vi "Convert RAWDATA_Denis.vi"(0 "Detector in":refnum<class "Detector.lvclass">, 1 "I channel":sgl[][](array[numeric]), 3 "WCM_values IN":sgl[](array[numeric]), 4 "II channel":sgl[][](array[numeric]), 5 "error in (no error)":errorcluster, 6 "# of scan":i32, 7 "All?":bool=TRUE, 10 "repump_limits":T1, 11 "repump_correction":bool, 12 "I channel seq IN":cluster{"BG":sgl[], "Ie":sgl[], "I0":sgl[]}[](array[cluster]), 13 "II channel seq IN":cluster{"BG":sgl[], "Ie":sgl[], "I0":sgl[]}[](array[cluster])) -> (14 "Detector out":refnum<class "Detector.lvclass">, 15 "I channel seq":cluster{"BG":sgl[], "Ie":sgl[], "I0":sgl[]}[](array[cluster]), 17 "WCM_correction_coff":sgl[](array[numeric]), 18 "II channel seq":cluster{"BG":sgl[], "Ie":sgl[], "I0":sgl[]}[](array[cluster]), 19 "error out":errorcluster)   [LabVIEW 2020, in "Detector.lvclass"]
uses:
  Detector.lvclass
  <userlib>/_OpenG.lib/array/array.llb/Search 1D Array (SGL)__ogtk.vi
  dependecies/globalVarII.vi
  dependecies/ControlsVIs/Clusters-def/Def_repump_limits.ctl
  Oscilloscope/Oscilloscope.lvclass
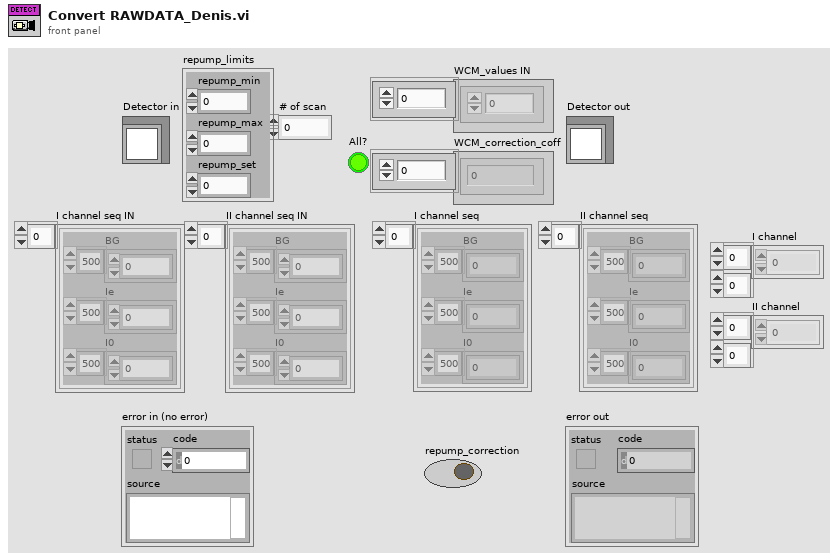
[diagram p1: front panel]
types:
  T1 = typedef "Oscilloscope.lvclass/Def_repump_limits.ctl" = cluster{"repump_min":dbl, "repump_max":dbl, "repump_set":dbl}
  T2 = typedef "Control-Client.lvclass/Controls-refs_CLIENT.ctl" = cluster{"ON/OFF Cool":refnum<vi>, "Save spectra":refnum<vi>, "Read detector":refnum<vi>, "# scans":refnum<vi>, "BG-level":refnum<vi>, "Set T":refnum<vi>, "Termometer":refnum<vi>, "Spectra":refnum<vi>, "Error Meter_ref":refnum<vi>, "OD graph":refnum<vi>, "from_pixel":refnum<vi>, "to_pixel":refnum<vi>, "threshold_ref_channel":refnum<vi>, "value":refnum<vi>, "python session":refnum<vi>, "ref h5_file":T3, "distance":refnum<vi>}
  T3 = typedef "hid_t.ctl" = i64
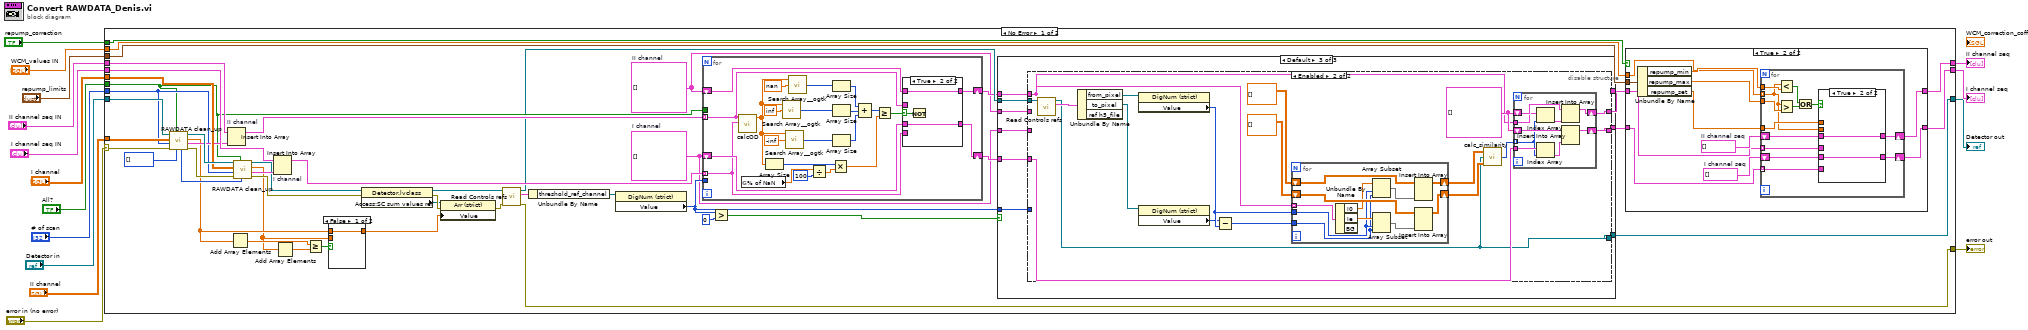
[diagram p0: block diagram]
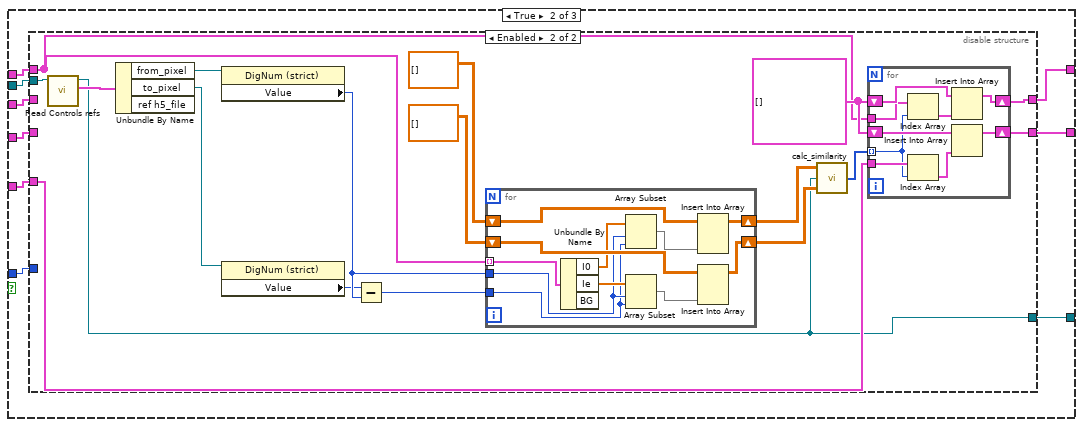
[diagram p3: hidden frame]
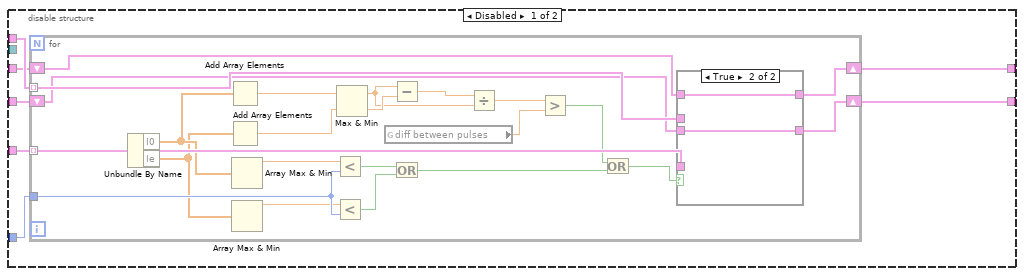
[diagram p4: hidden frame]
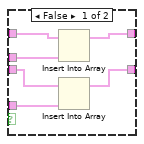
[diagram p5: hidden frame]
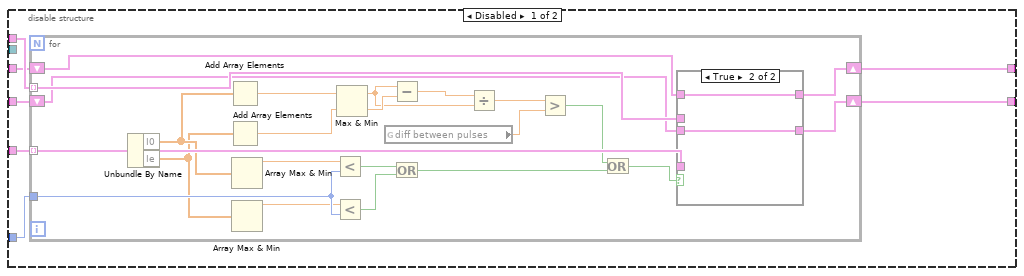
[diagram p6: hidden frame]
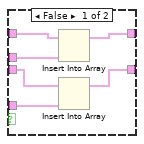
[diagram p7: hidden frame]
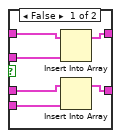
[diagram p8: hidden frame]
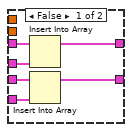
[diagram p11: hidden frame]
diagram:
  n1 = case shown="No Error" "error in (no error)" {
    selector: "error in (no error)" -> [w55 w306]
    tunnel: [w16 w307] -> w12
    tunnel: "Detector in" -> [w54 w307]
    tunnel: [w17 w306] -> w11
    tunnel: [w62 w305] -> w15
    tunnel: [w61 w304] -> w14
    tunnel: "II channel seq IN" -> [w60 w305]
    tunnel: "I channel seq IN" -> [w59 w304]
    tunnel: "WCM_values IN" -> [w58 _]
    tunnel: "I channel" -> [w44 _]
    tunnel: "II channel" -> [w46 _]
    tunnel: "repump_correction" -> [w57 _]
    tunnel: "repump_limits" -> [w56 _]
    tunnel: "All?" -> [w30 _]
    tunnel: "# of scan" -> [w37 _]
    frame No Error {
      w20 = cluster{"BG":sgl[], "Ie":sgl[], "I0":sgl[]}[] []  # II channel
      w21 = cluster{"BG":sgl[], "Ie":sgl[], "I0":sgl[]}[] []  # I channel
      n2 = call "RAWDATA clean_up.vi"("BG index IN"=i32[] [], "All?"=w30, "error in (no error)"=w55, "# of scan"=w37, "channel"=w46, "Detector in"=w54) -> ("error out"=w48:errorcluster, "channel seq"=w42:cluster{"BG":i32[], "Ie":i32[], "I0":i32[]}[], "SC values"=w38:sgl[], "Detector out"=w47:refnum<class "Detector.lvclass">, "BG indexes"=w45:i32[])  [unwired: 1 in]
      n3 = Insert Into Array "II channel"(array=w60, new element=w42) -> (w34:cluster{"BG":sgl[], "Ie":sgl[], "I0":sgl[]}[])  [unwired: 1 in]
      n4 = Add Array Elements(numeric array=w38) -> (sum=w51:sgl)
      n5 = call "RAWDATA clean_up.vi"("BG index IN"=w45, "All?"=w30, "error in (no error)"=w48, "# of scan"=w37, "channel"=w44, "Detector in"=w47) -> ("error out"=w40:errorcluster, "channel seq"=w43:cluster{"BG":i32[], "Ie":i32[], "I0":i32[]}[], "SC values"=w31:sgl[], "Detector out"=w41:refnum<class "Detector.lvclass">)  [unwired: 1 in, 1 out]
      n6 = Insert Into Array "I channel"(array=w59, new element=w43) -> (w35:cluster{"BG":sgl[], "Ie":sgl[], "I0":sgl[]}[])  [unwired: 1 in]
      n7 = Add Array Elements(numeric array=w31) -> (sum=w50:sgl)
      n8 = Greater Or Equal?(x=w51, y=w50) -> (x >= y?=w49:bool)
      n9 = case shown="False" w49 {
        tunnel: w38 -> [w268 _]
        tunnel: [w268 w269] -> w39
        tunnel: w31 -> [_ w269]
        frame False {
        }
        frame True {
        }
      }
      n10 = property class="Detector.lvclass"(reference=w41, error in=w40) -> (reference out=w28:refnum<class "Detector.lvclass">, error out=w53:errorcluster, "Access:SC sum values ref"=w52:refnum<vi>)
      n11 = property class="Arr (strict)"(reference=w52, error in=w53, "Value"=w39) -> (error out=w29:errorcluster)  [unwired: 1 out]
      n12 = call "Read Controls refs.vi"("error in (no error)"=w29, "Detector in"=w28) -> ("error out"=w17:errorcluster, "Controls refs"=w27:T2, "Detector out"=w24:refnum<class "Detector.lvclass">)  [unwired: 7 in]
      n13 = Unbundle By Name(w27) -> ("threshold_ref_channel"=w26:refnum<vi>)
      n14 = property class="DigNum (strict)"(reference=w26) -> ("Value"=w25:i32)  [unwired: 1 in, 2 out]
      n15 = for {
        tunnel: w35 -> [w238] mode=indexing
        tunnel: w34 -> [w248] mode=indexing
        shift-right: [w236] -> w22
        shift-left: w21 -> [w250]
        shift-right: [w237] -> w23
        shift-left: w20 -> [w249]
        tunnel: w30 -> [_]
        tunnel: w25 -> [_]
        n16 = call "calcOD.vi"("channel I"=w238, "channel 2"=w248) -> ("OD"=w256:sgl[])  [unwired: 3 in, 6 out]
        n17 = global read "globalVarII.vi" "% of NaN"() -> (w246:sgl)
        n18 = Array Size(array=w256) -> (size(s)=w255:i32)
        n19 = call-poly <userlib>:"Search Array__ogtk.vi"("Array"=w256, "Element Data"=sgl inf) -> ("Indices of Elements"=w254:i32[])  [unwired: 7 in]
        n20 = call-poly <userlib>:"Search Array__ogtk.vi"("Array"=w256, "Element Data"=sgl -inf) -> ("Indices of Elements"=w253:i32[])  [unwired: 7 in]
        n21 = call-poly <userlib>:"Search Array__ogtk.vi"("Array"=w256, "Element Data"=sgl nan) -> ("Indices of Elements"=w257:i32[])  [unwired: 7 in]
        n22 = Divide(x=w246, y=100) -> (x/y=w247:sgl)
        n23 = Multiply(x=w255, y=w247) -> (x*y=w240:sgl)
        n24 = Array Size(array=w257) -> (size(s)=w244:i32)
        n25 = Array Size(array=w254) -> (size(s)=w243:i32)
        n26 = Array Size(array=w253) -> (size(s)=w242:i32)
        n27 = Compound Arithmetic op=ADD(w244, w243, w242) -> (w241:i32)
        n28 = Greater Or Equal?(x=w241, y=w240) -> (x >= y?=w239:bool)
        n29 = case shown="True" w239 {
          selector: w239 -> [_ w265]
          tunnel: w250 -> [w264 w266]
          tunnel: w238 -> [w263 _]
          tunnel: [w262 w266] -> w236
          tunnel: [w261 w267] -> w237
          tunnel: w249 -> [w260 w267]
          tunnel: w248 -> [w259 _]
          frame False {
            n30 = Insert Into Array(array=w260, new element=w259) -> (w261:cluster{"BG":sgl[], "Ie":sgl[], "I0":sgl[]}[])  [unwired: 1 in]
            n31 = Insert Into Array(array=w264, new element=w263) -> (w262:cluster{"BG":sgl[], "Ie":sgl[], "I0":sgl[]}[])  [unwired: 1 in]
          }
          frame True {
            n32 = Not(x=w265) -> ()  [unwired: 1 out]
          }
        }
      }
      n33 = Greater?(x=w25, y=0) -> (0:w18:bool)
      n34 = case w18 {
        tunnel: [w65 w70 w155] -> w32
        tunnel: w23 -> [w65 w74 w159]
        tunnel: w22 -> [w64 w73 w158]
        tunnel: [w64 w69 w154] -> w33
        tunnel: w21 -> [_ w72 w157]
        tunnel: w20 -> [_ w71 w156]
        tunnel: w25 -> [_ w68 w153]
        tunnel: w24 -> [w63 w67 w152]
        tunnel: [w63 w66 w151] -> w16
        frame False {
        }
        frame True {
          n35 = disable-structure shown="Enabled" {
            disable-tunnel: w74 -> [w81 w113]
            disable-tunnel: w73 -> [w80 w127]
            disable-tunnel: w72 -> [w79 _]
            disable-tunnel: w71 -> [w78 _]
            disable-tunnel: [w77 w124] -> w70
            disable-tunnel: [w76 w126] -> w69
            disable-tunnel: w68 -> [w75 _]
            disable-tunnel: w67 -> [_ w120]
            disable-tunnel: [_ w114] -> w66
            frame Disabled {
              n36 = for {
                tunnel: w81 -> [w100] mode=indexing
                tunnel: w80 -> [w99] mode=indexing
                shift-right: [w97] -> w76
                shift-left: w79 -> [w98]
                shift-right: [w101] -> w77
                shift-left: w78 -> [w102]
                tunnel: w75 -> [w96]
                n37 = Unbundle By Name(w99) -> ("I0"=w91:sgl[], "Ie"=w90:sgl[])
                n38 = Add Array Elements(numeric array=w91) -> (sum=w89:sgl)
                n39 = Add Array Elements(numeric array=w90) -> (sum=w88:sgl)
                n40 = Array Max & Min(array=w91) -> (max value=w93:sgl)  [unwired: 3 out]
                n41 = Array Max & Min(array=w90) -> (max value=w92:sgl)  [unwired: 3 out]
                n42 = Less?(x=w93, y=w96) -> (x < y?=w103:bool)
                n43 = Less?(x=w92, y=w96) -> (x < y?=w104:bool)
                n44 = Max & Min(x=w89, y=w88) -> (max(x,y)=w85:sgl, min(x,y)=w87:sgl)
                n45 = global read "globalVarII.vi" "diff between pulses"() -> (w82:dbl)
                n46 = Subtract(x=w85, y=w87) -> (x-y=w86:sgl)
                n47 = Or(x=w103, y=w104) -> (x .or. y?=w95:bool)
                n48 = Divide(x=w86, y=w85) -> (x/y=w84:sgl)
                n49 = Greater?(x=w84, y=w82) -> (0:w83:bool)
                n50 = Or(x=w83, y=w95) -> (x .or. y?=w94:bool)
                n51 = case shown="True" w94 {
                  tunnel: w102 -> [w110 w112]
                  tunnel: [w109 w112] -> w101
                  tunnel: w100 -> [w108 _]
                  tunnel: w99 -> [w107 _]
                  tunnel: w98 -> [w106 w111]
                  tunnel: [w105 w111] -> w97
                  frame False {
                    n52 = Insert Into Array(array=w110, new element=w108) -> (w109:cluster{"BG":sgl[], "Ie":sgl[], "I0":sgl[]}[])  [unwired: 1 in]
                    n53 = Insert Into Array(array=w106, new element=w107) -> (w105:cluster{"BG":sgl[], "Ie":sgl[], "I0":sgl[]}[])  [unwired: 1 in]
                  }
                  frame True {
                  }
                }
              }
            }
            frame Enabled {
              w125 = cluster{"BG":sgl[], "Ie":sgl[], "I0":sgl[]}[] [] ("I channel")
              n54 = call "Read Controls refs.vi"("Detector in"=w120) -> ("Controls refs"=w119:T2, "Detector out"=w114:refnum<class "Detector.lvclass">)  [unwired: 8 in, 1 out]
              n55 = Unbundle By Name(w119) -> ("from_pixel"=w118:refnum<vi>, "to_pixel"=w117:refnum<vi>)  [unwired: 1 out]
              n56 = property class="DigNum (strict)"(reference=w118) -> ("Value"=w116:i32)  [unwired: 1 in, 2 out]
              n57 = property class="DigNum (strict)"(reference=w117) -> ("Value"=w115:i32)  [unwired: 1 in, 2 out]
              n58 = Subtract(x=w115, y=w116) -> (x-y=w121:i32)
              n59 = for {
                tunnel: w113 -> [w150] mode=indexing
                shift-right: [w148] -> w128
                shift-left: dbl[][] [] -> [w149]
                shift-right: [w146] -> w122
                shift-left: dbl[][] [] -> [w147]
                tunnel: w116 -> [w141]
                tunnel: w121 -> [w140]
                n60 = Unbundle By Name(w150) -> ("I0"=w143:sgl[], "Ie"=w145:sgl[])  [unwired: 1 out]
                n61 = Array Subset(array=w143, index=w141, length=w140) -> (w142:sgl[])
                n62 = Array Subset(array=w145, index=w141, length=w140) -> (w144:sgl[])
                n63 = Insert Into Array(array=w149, new element=w142) -> (w148:dbl[][])  [unwired: 2 in]
                n64 = Insert Into Array(array=w147, new element=w144) -> (w146:dbl[][])  [unwired: 2 in]
              }
              n65 = call "calc_similarity.vi"("data2"=w122, "Detector in"=w114, "data1"=w128) -> ("similarity out"=w123:i32[])
              n66 = for {
                tunnel: w127 -> [w139]
                shift-right: [w136] -> w126
                shift-left: w125 -> [w137]
                shift-right: [w135] -> w124
                shift-left: w125 -> [w134]
                tunnel: w113 -> [w133]
                tunnel: w123 -> [w131] mode=indexing
                n67 = Index Array(array=w133, index=w131) -> (element=w132:cluster{"BG":sgl[], "Ie":sgl[], "I0":sgl[]})
                n68 = Index Array(array=w139, index=w131) -> (element=w138:cluster{"BG":sgl[], "Ie":sgl[], "I0":sgl[]})
                n69 = Insert Into Array(array=w134, new element=w132) -> (w135:cluster{"BG":sgl[], "Ie":sgl[], "I0":sgl[]}[])  [unwired: 1 in]
                n70 = Insert Into Array(array=w137, new element=w138) -> (w136:cluster{"BG":sgl[], "Ie":sgl[], "I0":sgl[]}[])  [unwired: 1 in]
              }
            }
          }
        }
        frame Default {
          n71 = disable-structure shown="Enabled" {
            disable-tunnel: w159 -> [w166 w198]
            disable-tunnel: w158 -> [w165 w212]
            disable-tunnel: w157 -> [w164 _]
            disable-tunnel: w156 -> [w163 _]
            disable-tunnel: [w162 w209] -> w155
            disable-tunnel: [w161 w211] -> w154
            disable-tunnel: w153 -> [w160 _]
            disable-tunnel: w152 -> [_ w205]
            disable-tunnel: [_ w199] -> w151
            frame Disabled {
              n72 = for {
                tunnel: w166 -> [w185] mode=indexing
                tunnel: w165 -> [w184] mode=indexing
                shift-right: [w182] -> w161
                shift-left: w164 -> [w183]
                shift-right: [w186] -> w162
                shift-left: w163 -> [w187]
                tunnel: w160 -> [w181]
                n73 = Unbundle By Name(w184) -> ("I0"=w176:sgl[], "Ie"=w175:sgl[])
                n74 = Add Array Elements(numeric array=w176) -> (sum=w174:sgl)
                n75 = Add Array Elements(numeric array=w175) -> (sum=w173:sgl)
                n76 = Array Max & Min(array=w176) -> (max value=w178:sgl)  [unwired: 3 out]
                n77 = Array Max & Min(array=w175) -> (max value=w177:sgl)  [unwired: 3 out]
                n78 = Less?(x=w178, y=w181) -> (x < y?=w188:bool)
                n79 = Less?(x=w177, y=w181) -> (x < y?=w189:bool)
                n80 = Max & Min(x=w174, y=w173) -> (max(x,y)=w170:sgl, min(x,y)=w172:sgl)
                n81 = global read "globalVarII.vi" "diff between pulses"() -> (w167:dbl)
                n82 = Subtract(x=w170, y=w172) -> (x-y=w171:sgl)
                n83 = Or(x=w188, y=w189) -> (x .or. y?=w180:bool)
                n84 = Divide(x=w171, y=w170) -> (x/y=w169:sgl)
                n85 = Greater?(x=w169, y=w167) -> (0:w168:bool)
                n86 = Or(x=w168, y=w180) -> (x .or. y?=w179:bool)
                n87 = case shown="True" w179 {
                  tunnel: w187 -> [w195 w197]
                  tunnel: [w194 w197] -> w186
                  tunnel: w185 -> [w193 _]
                  tunnel: w184 -> [w192 _]
                  tunnel: w183 -> [w191 w196]
                  tunnel: [w190 w196] -> w182
                  frame False {
                    n88 = Insert Into Array(array=w195, new element=w193) -> (w194:cluster{"BG":sgl[], "Ie":sgl[], "I0":sgl[]}[])  [unwired: 1 in]
                    n89 = Insert Into Array(array=w191, new element=w192) -> (w190:cluster{"BG":sgl[], "Ie":sgl[], "I0":sgl[]}[])  [unwired: 1 in]
                  }
                  frame True {
                  }
                }
              }
            }
            frame Enabled {
              w210 = cluster{"BG":sgl[], "Ie":sgl[], "I0":sgl[]}[] [] ("I channel")
              n90 = call "Read Controls refs.vi"("Detector in"=w205) -> ("Controls refs"=w204:T2, "Detector out"=w199:refnum<class "Detector.lvclass">)  [unwired: 8 in, 1 out]
              n91 = Unbundle By Name(w204) -> ("from_pixel"=w203:refnum<vi>, "to_pixel"=w202:refnum<vi>)  [unwired: 1 out]
              n92 = property class="DigNum (strict)"(reference=w203) -> ("Value"=w201:i32)  [unwired: 1 in, 2 out]
              n93 = property class="DigNum (strict)"(reference=w202) -> ("Value"=w200:i32)  [unwired: 1 in, 2 out]
              n94 = Subtract(x=w200, y=w201) -> (x-y=w206:i32)
              n95 = for {
                tunnel: w198 -> [w235] mode=indexing
                shift-right: [w233] -> w213
                shift-left: dbl[][] [] -> [w234]
                shift-right: [w231] -> w207
                shift-left: dbl[][] [] -> [w232]
                tunnel: w201 -> [w226]
                tunnel: w206 -> [w225]
                n96 = Unbundle By Name(w235) -> ("I0"=w228:sgl[], "Ie"=w230:sgl[])  [unwired: 1 out]
                n97 = Array Subset(array=w228, index=w226, length=w225) -> (w227:sgl[])
                n98 = Array Subset(array=w230, index=w226, length=w225) -> (w229:sgl[])
                n99 = Insert Into Array(array=w234, new element=w227) -> (w233:dbl[][])  [unwired: 2 in]
                n100 = Insert Into Array(array=w232, new element=w229) -> (w231:dbl[][])  [unwired: 2 in]
              }
              n101 = call "calc_similarity.vi"("data2"=w207, "Detector in"=w199, "data1"=w213) -> ("similarity out"=w208:i32[])
              n102 = for {
                tunnel: w212 -> [w224]
                shift-right: [w221] -> w211
                shift-left: w210 -> [w222]
                shift-right: [w220] -> w209
                shift-left: w210 -> [w219]
                tunnel: w198 -> [w218]
                tunnel: w208 -> [w216] mode=indexing
                n103 = Index Array(array=w218, index=w216) -> (element=w217:cluster{"BG":sgl[], "Ie":sgl[], "I0":sgl[]})
                n104 = Index Array(array=w224, index=w216) -> (element=w223:cluster{"BG":sgl[], "Ie":sgl[], "I0":sgl[]})
                n105 = Insert Into Array(array=w219, new element=w217) -> (w220:cluster{"BG":sgl[], "Ie":sgl[], "I0":sgl[]}[])  [unwired: 1 in]
                n106 = Insert Into Array(array=w222, new element=w223) -> (w221:cluster{"BG":sgl[], "Ie":sgl[], "I0":sgl[]}[])  [unwired: 1 in]
              }
            }
          }
        }
      }
      n107 = case shown="True" w57 {
        tunnel: [w271 w275] -> w62
        tunnel: w32 -> [w271 w277]
        tunnel: [w270 w276] -> w61
        tunnel: w33 -> [w270 w278]
        tunnel: w58 -> [_ w274]
        tunnel: w56 -> [_ w273]
        frame False {
        }
        frame True {
          w281 = cluster{"BG":i32[], "Ie":i32[], "I0":i32[]}[] []  # II channel seq
          w282 = cluster{"BG":i32[], "Ie":i32[], "I0":i32[]}[] []  # I channel seq
          n108 = Unbundle By Name(w273) -> ("repump_min"=w280:dbl, "repump_max"=w279:dbl, "repump_set"=w272:dbl)
          n109 = for {
            tunnel: w279 -> [w294]
            tunnel: w280 -> [w295]
            shift-right: [w288] -> w275
            shift-left: w281 -> [w287]
            shift-right: [w289] -> w276
            shift-left: w282 -> [w290]
            tunnel: w278 -> [w286] mode=indexing
            tunnel: w277 -> [w285] mode=indexing
            tunnel: w274 -> [w283] mode=indexing
            tunnel: w272 -> [w284]
            n110 = Less?(x=w283, y=w295) -> (x < y?=w293:bool)
            n111 = Greater?(x=w283, y=w294) -> (0:w292:bool)
            n112 = Or(x=w293, y=w292) -> (x .or. y?=w291:bool)
            n113 = case shown="True" w291 {
              tunnel: w290 -> [w301 w303]
              tunnel: [w300 w303] -> w289
              tunnel: [w298 w302] -> w288
              tunnel: w287 -> [w299 w302]
              tunnel: w286 -> [w297 _]
              tunnel: w285 -> [w296 _]
              tunnel: w284 -> [_ _]
              tunnel: w283 -> [_ _]
              frame False {
                n114 = Insert Into Array(array=w299, new element=w296) -> (w298:cluster{"BG":i32[], "Ie":i32[], "I0":i32[]}[])  [unwired: 1 in]
                n115 = Insert Into Array(array=w301, new element=w297) -> (w300:cluster{"BG":i32[], "Ie":i32[], "I0":i32[]}[])  [unwired: 1 in]
              }
              frame True {
              }
            }
          }
        }
      }
    }
    frame Error {
    }
  }
  "error out" <- w11
  "Detector out" <- w12
  "II channel seq" <- w15
  "I channel seq" <- w14
